vi "Launch Example Dialog.vi"() -> ()   [LabVIEW 2020]
uses:
  <vilib>/ActorFramework/LastAck/Last Ack.lvclass
  Example Configuration Dialog.lvclass
  C:/Program Files/National Instruments/LabVIEW 2020/vi.lib/ActorFramework/Actor/Actor.lvclass
  <vilib>/ActorFramework/Message Queue/Message Queue.lvclass/Message Queue.ctl
  <vilib>/ActorFramework/Message Dequeuer/Message Dequeuer.lvclass/Message Dequeuer.ctl
  <vilib>/ActorFramework/LastAck/Last Ack.lvclass/Last Ack.ctl
  <vilib>/ActorFramework/Message Priority Queue/Priority Dequeue.vi
  <vilib>/ActorFramework/Actor/Actor.lvclass
  <vilib>/ActorFramework/Message Queue/Message Queue.lvclass
  <vilib>/ActorFramework/Message Dequeuer/Message Dequeuer.lvclass
  Configuration.lvclass
panel:
  in  "Stop Button":bool
  out "Configuration File Path Parameters Saved To: (will be the same as above unless invalid or no path was given)":path
  out "error IO":errorcluster
  in  "Configuration File Path to Load":path
  # "Run this test VI to launch the configuration dialog to act upon this file:"
  # "Stopping this actor requires firing the user-event that terminates any blocking event cases in the actor methods. This is\nonly necessary if you do not want the dialog to be modal."
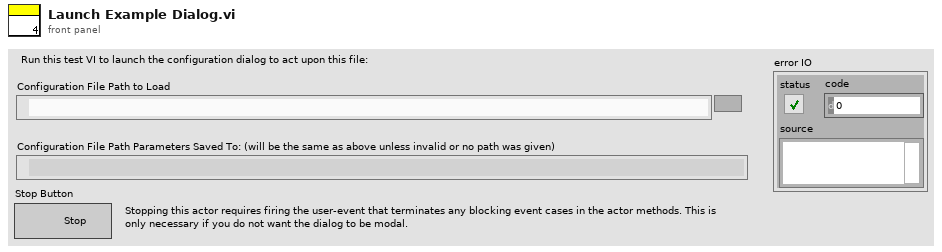
[diagram p1: front panel]
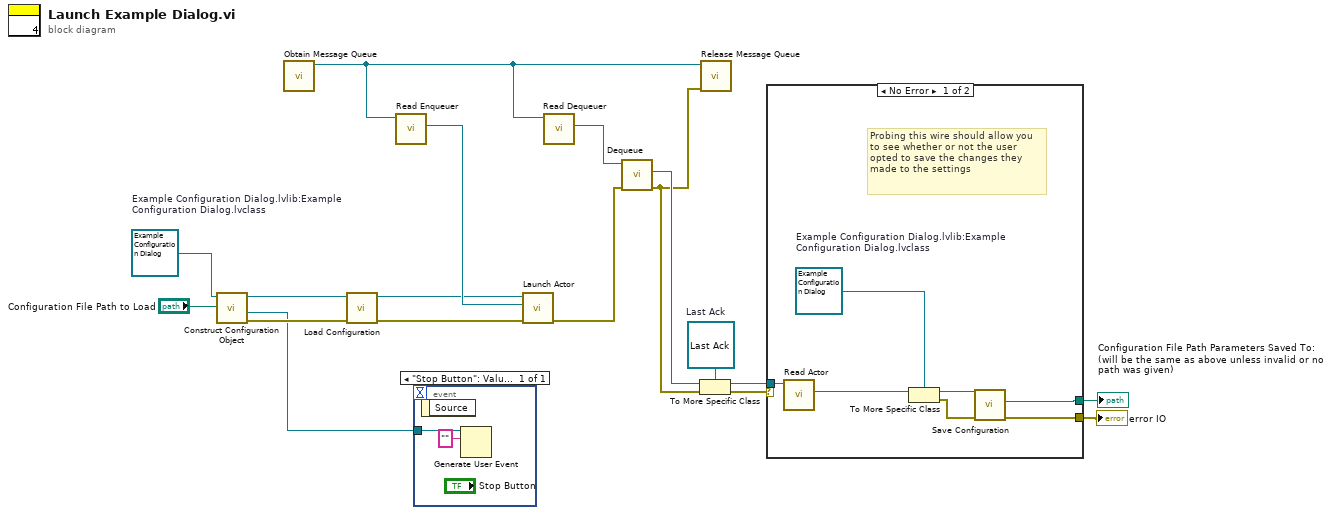
[diagram p0: block diagram]
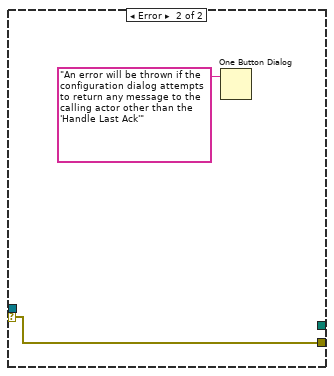
[diagram p2: hidden frame]
diagram:
  w6 = refnum<class "Example Configuration Dialog.lvclass"> refnum  # Example Configuration Dialog.lvlib:Example Configuration Dialog.lvclass
  w11 = refnum<class "Last Ack.lvclass"> refnum  # Last Ack
  n1 = call "Construct Configuration Object.vi"("Configuration File Path"="Configuration File Path to Load", "Configuration in"=w6) -> ("error out"=w8:errorcluster, "Stop Event"=w3:refnum<user-event>, "Configuration out"=w17:refnum<class "Example Configuration Dialog.lvclass">)  [unwired: 6 in, 1 out]
  n2 = call <vilib>:"Obtain Message Queue.vi"() -> ("Message Queue"=w15:refnum<class "Message Queue.lvclass">)  [unwired: 10 in, 1 out]
  n3 = call "Load Configuration.vi"("error in (no error)"=w8, "Configuration in"=w17) -> ("error out"=w7:errorcluster, "Configuration out"=w1:refnum<class "Example Configuration Dialog.lvclass">)  [unwired: 7 in, 1 out]
  n4 = call <vilib>:"Read Enqueuer.vi"("Message Queue"=w15) -> ("Message Enqueuer"=w18:refnum<class "Message Enqueuer.lvclass">)  [unwired: 10 in]
  n5 = event shown="[0] \"Stop Button\": Value Change" {
    selector: _ -> [_]
    dyn-events: _ -> [_]
    timeout: _ -> [_]
    tunnel: w3 -> [w20]
    event "Stop Button": Value Change {
      n6 = event-data() -> ()  [unwired: 1 in, 1 out]
      n7 = Generate User Event(user event=w20, event data cluster="" ("event data")) -> ()  [unwired: 2 in, 2 out]
    }
  }
  n8 = call <vilib>:"Launch Actor.vi"("error in (no error)"=w7, "Actor-to-Caller Enqueuer"=w18, "Actor"=w1) -> ("error out"=w13:errorcluster)  [unwired: 7 in, 1 out]
  n9 = call <vilib>:"Read Dequeuer.vi"("Message Queue"=w15) -> ("Message Dequeuer"=w14:refnum<class "Message Dequeuer.lvclass">)  [unwired: 10 in]
  n10 = call <vilib>:"Dequeue.vi"("error in (no error)"=w13, "Message Dequeuer in"=w14) -> ("error out"=w2:errorcluster, "Message"=w12:refnum<class "Message.lvclass">)  [unwired: 5 in, 3 out]
  n11 = To More Specific Class(target class=w11, reference=w12, error in=w2) -> (specific class reference=w10:refnum<class "Last Ack.lvclass">, error out=w9:errorcluster)
  n12 = call <vilib>:"Release Message Queue.vi"("error in (no error)"=w2, "Message Queue"=w15) -> ()  [unwired: 8 in, 2 out]
  n13 = case shown="No Error" w9 {
    selector: w9 -> [_ w28]
    tunnel: w10 -> [w27 _]
    tunnel: [w24 w28] -> w5
    tunnel: [w23 _] -> w4
    frame No Error {
      w22 = refnum<class "Example Configuration Dialog.lvclass"> refnum  # Example Configuration Dialog.lvlib:Example Configuration Dialog.lvclass
      # "Probing this wire should allow you to see whether or not the user opted to save the changes they made to the settings"
      n14 = call <vilib>:"Read Actor.vi"("Last Ack"=w27) -> ("Actor"=w26:refnum<class "Actor.lvclass">)  [unwired: 10 in]
      n15 = To More Specific Class(target class=w22, reference=w26) -> (specific class reference=w21:refnum<class "Example Configuration Dialog.lvclass">, error out=w25:errorcluster)  [unwired: 1 in]
      n16 = call "Save Configuration.vi"("error in (no error)"=w25, "Configuration in"=w21) -> ("error out"=w24:errorcluster, "file path"=w23:path)  [unwired: 7 in, 1 out]
    }
    frame Error {
      n17 = One Button Dialog(message="An error will be thrown if the configuration dialog attempts to return any message to the calling actor other than the 'Handle Last Ack'") -> ()  [unwired: 1 in, 1 out]
    }
  }
  "error IO" <- w5
  "Configuration File Path Parameters Saved To: (will be the same as above unless invalid or no path was given)" <- w4
